vi "settings.vi"(7 "LabVIEW Web Service Request":refnum<class "Web Request.lvclass">, 9 "password":string, 10 "reservation_id":string, 11 "context_id":string) -> (3 "response":string)   [LabVIEW 2013]
uses:
  <vilib>/wsapi/Web Request.lvclass
  <vilib>/Utility/config.llb/Read Key (String).vi
  <vilib>/Utility/config.llb/Write Key (String).vi
  <vilib>/Utility/config.llb/NI_LVConfig.lvlib
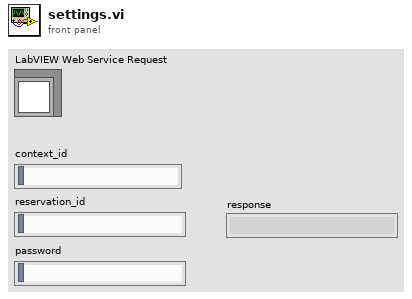
[diagram p1: front panel]
types:
  T1 = typedef "NI_LVConfig.lvlib/Config Data RefNum.ctl" = refnum<k1>
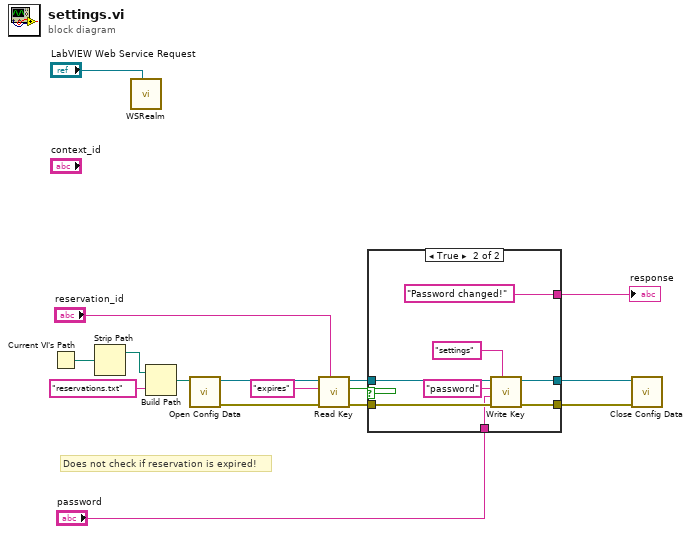
[diagram p0: block diagram]
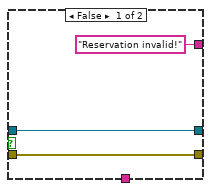
[diagram p2: hidden frame]
diagram:
  # "Does not check if reservation is expired!"
  n1 = Current VI's Path() -> (path=w15:path)
  n2 = Strip Path(path=w15) -> (stripped path=w14:path)  [unwired: 1 out]
  n3 = call "WSRealm.vi"("LabVIEW Web Service Request"="LabVIEW Web Service Request") -> ()  [unwired: 11 in]
  n4 = Build Path(base path=w14, name or relative path="reservations.txt") -> (appended path=w12:path)
  n5 = call <vilib>:"Open Config Data.vi"("configuration file path"=w12) -> ("error out"=w9:errorcluster, "refnum"=w10:T1)  [unwired: 8 in, 1 out]
  n6 = call-poly <vilib>:"Read Key.vi"("section"="reservation_id", "error in (no error)"=w9, "key"="expires", "refnum"=w10) -> ("error out"=w5:errorcluster, "found?"=w7:bool, "refnum out"=w6:T1)  [unwired: 4 in, 1 out]
  n7 = case shown="True" w7 {
    tunnel: w6 -> [w19 w27]
    tunnel: w5 -> [w18 w26]
    tunnel: ["Reservation invalid!" ("response") "Password changed!" ("response")] -> w4
    tunnel: [w19 w22] -> w3
    tunnel: [w18 w21] -> w2
    tunnel: "password" -> [_ w20]
    frame False {
    }
    frame True {
      n8 = call-poly <vilib>:"Write Key.vi"("section"="settings", "error in (no error)"=w26, "value"=w20, "key"="password", "refnum"=w27) -> ("error out"=w21:errorcluster, "refnum out"=w22:T1)  [unwired: 4 in, 1 out]
    }
  }
  "response" <- w4
  n9 = call <vilib>:"Close Config Data.vi"("error in (no error)"=w2, "refnum"=w3) -> ()  [unwired: 8 in, 2 out]
